vi "Read Metadata from TDMS.vi"(8 "error in (no error)":errorcluster, 11 "file path":path) -> (0 "error out":errorcluster, 1 "wiring config":string[][](array[string]), 2 "scan info":T1)   [LabVIEW 2016]
uses:
  subvi/ctl/Scan Info -- Cluster.ctl
panel:
  out "priorities":string[](array[string])
  out "starts":dbl[](array[numeric])
  out "ends":dbl[](array[numeric])
  out "steps":dbl[](array[numeric])
  out "scan names":string[](array[string])
  out "property values":variant[](array[variant])
  out "property names":string[](array[string])
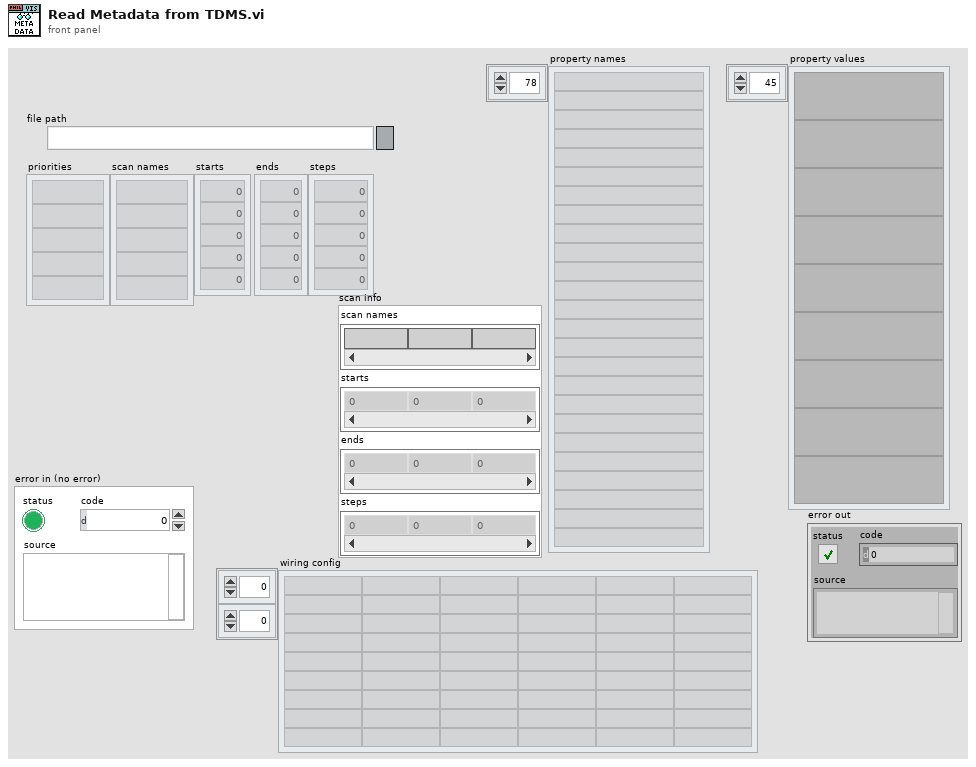
[diagram p1: front panel]
types:
  T1 = typedef "Scan Info -- Cluster.ctl" = cluster{"scan names":string[], "starts":dbl[], "ends":dbl[], "steps":dbl[]}
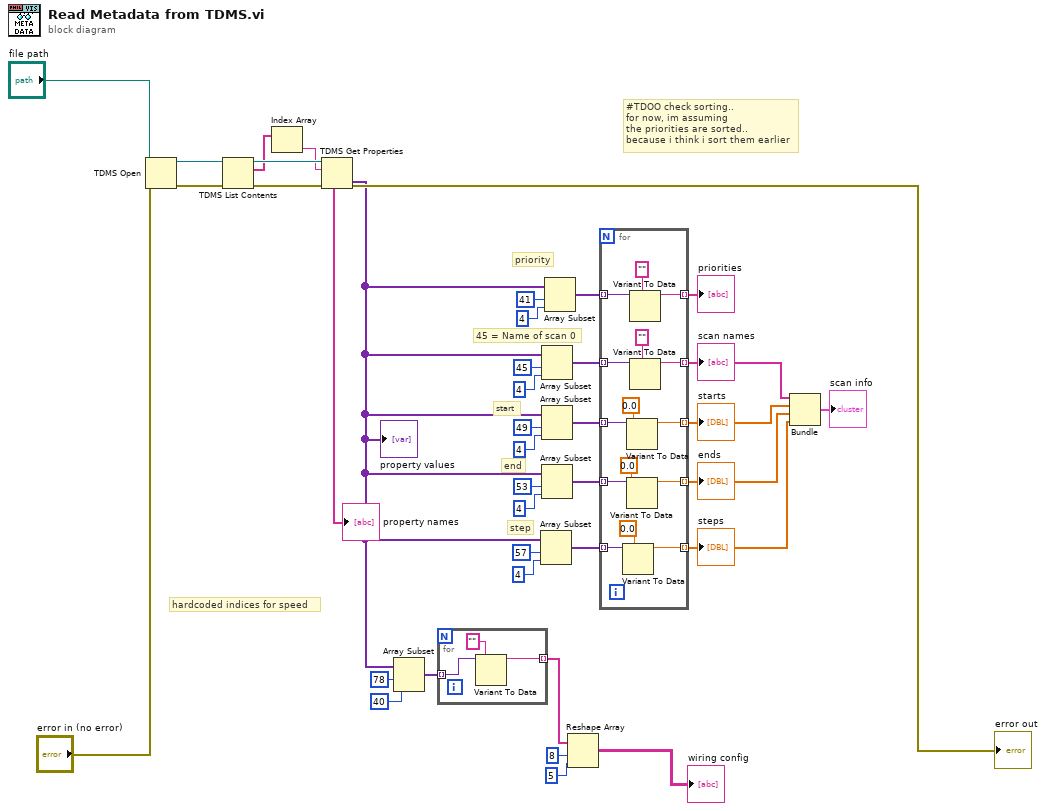
[diagram p0: block diagram]
diagram:
  # "#TDOO check sorting..\nfor now, im assuming \nthe priorities are sorted..\nbecause i think i sort them earlier"
  # "priority"
  # "step"
  # "end"
  # "start"
  # "45 = Name of scan 0"
  # "hardcoded indices for speed"
  n1 = TDMS Open(8:"error in (no error)", 11:"file path") -> (0:w36:errorcluster, 3:w35:refnum<k34>)  [unwired: 5 in]
  n2 = TDMS List Contents(4:w36, 7:w35) -> (0:w34:errorcluster, 2:w32:string[], 3:w33:refnum<k34>)  [unwired: 1 in, 1 out]
  n3 = Index Array(array=w32) -> (element=w31:string)  [unwired: 1 in]
  n4 = TDMS Get Properties(8:w34, 10:w31, 11:w33) -> (0:→"error out":errorcluster, 4:w1:variant[], 6:→"property names":string[])  [unwired: 3 in, 3 out]
  "property values" <- w1
  n5 = Array Subset(array=w1, index=78, length=40 ("index")) -> (w3:variant[])
  n6 = for {
    tunnel: w3 -> [w40] mode=indexing
    tunnel: [w42] -> w2 mode=indexing
    n7 = Variant To Data(type="", Variant=w40) -> (data=w42:string)  [unwired: 1 in, 1 out]
  }
  n8 = Array Subset(array=w1, index=57, length=4) -> (w21:variant[])
  n9 = Array Subset(array=w1, index=45, length=4) -> (w28:variant[])
  n10 = Array Subset(array=w1, index=49, length=4) -> (w19:variant[])
  n11 = Array Subset(array=w1, index=53, length=4) -> (w20:variant[])
  n12 = Array Subset(array=w1, index=41, length=4) -> (w16:variant[])
  n13 = Reshape Array(w2, 8 ("dimension size"), 5 ("dimension size")) -> (→"wiring config":string[][])
  n14 = for {
    tunnel: w28 -> [w56] mode=indexing
    tunnel: [w55] -> w14 mode=indexing
    tunnel: w21 -> [w51] mode=indexing
    tunnel: w20 -> [w50] mode=indexing
    tunnel: w19 -> [w49] mode=indexing
    tunnel: [w48] -> w13 mode=indexing
    tunnel: [w47] -> w12 mode=indexing
    tunnel: [w46] -> w11 mode=indexing
    tunnel: w16 -> [w44] mode=indexing
    tunnel: [w43] -> w15 mode=indexing
    n15 = Variant To Data(type=0.0, Variant=w51) -> (data=w46:dbl)  [unwired: 1 in, 1 out]
    n16 = Variant To Data(type=0.0, Variant=w49) -> (data=w48:dbl)  [unwired: 1 in, 1 out]
    n17 = Variant To Data(type=0.0, Variant=w50) -> (data=w47:dbl)  [unwired: 1 in, 1 out]
    n18 = Variant To Data(type="", Variant=w44) -> (data=w43:string)  [unwired: 1 in, 1 out]
    n19 = Variant To Data(type="", Variant=w56) -> (data=w55:string)  [unwired: 1 in, 1 out]
  }
  "scan names" <- w14
  "steps" <- w11
  "ends" <- w12
  "starts" <- w13
  "priorities" <- w15
  n20 = Bundle(w14, w13, w12, w11) -> (→"scan info":cluster{string[], dbl[], dbl[], dbl[]})  [unwired: 1 in]
